vi "Wait CAM.vi"(8 "error in (no error)":errorcluster, 10 "Numeric Control":u16, 11 "CCD in":refnum<class "CCD.lvclass">) -> (0 "error out":errorcluster, 3 "CCD out":refnum<class "CCD.lvclass">)   [LabVIEW 2018, in "CCD.lvclass"]
uses:
  CCD.lvclass
  CCD.lvclass/CCD.ctl
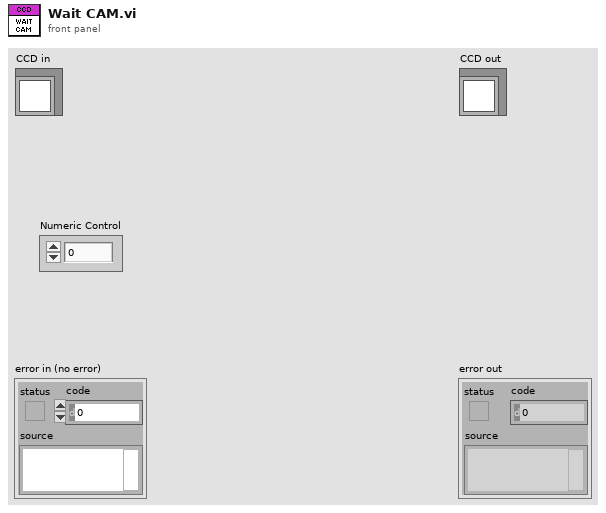
[diagram p1: front panel]
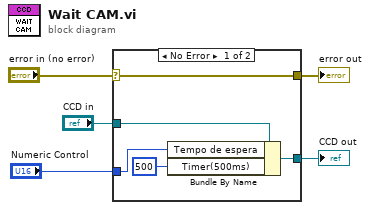
[diagram p0: block diagram]
diagram:
  n1 = case shown="No Error" "error in (no error)" {
    selector: "error in (no error)" -> [w10 w11]
    tunnel: [w10 w11] -> w3
    tunnel: [w8 w12] -> w2
    tunnel: "CCD in" -> [w9 w12]
    tunnel: "Numeric Control" -> [w6 _]
    frame No Error {
      n2 = Bundle By Name(cluster=w9, "Tempo de espera"=w6, "Timer(500ms)"=u16 500) -> (w8:refnum<class "CCD.lvclass">)
    }
    frame Error {
    }
  }
  "error out" <- w3
  "CCD out" <- w2
